vi "Write Interface Infos.vi"(8 "error in (no error)":errorcluster, 10 "Interface Infos":T1, 11 "Application in":refnum<class "Application.lvclass">) -> (0 "error out":errorcluster, 3 "Application out":refnum<class "Application.lvclass">)   [LabVIEW 2018, in "Application.lvclass"]
uses:
  Application.lvclass
  Application.lvclass/Application.ctl
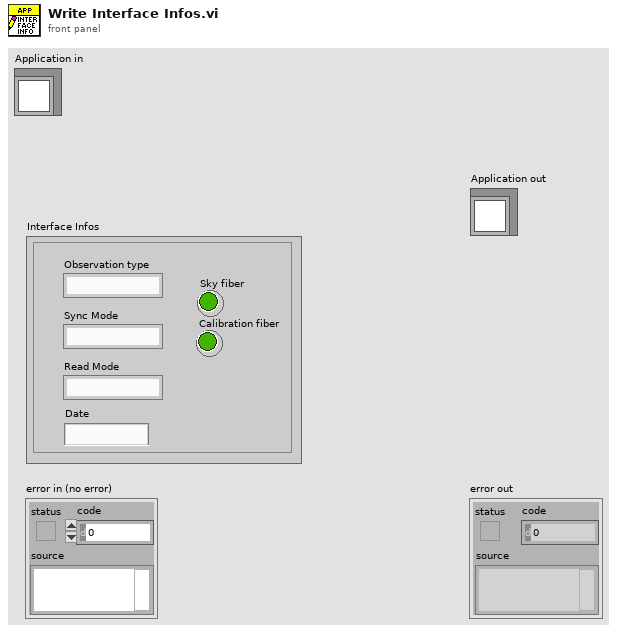
[diagram p1: front panel]
types:
  T1 = cluster{"Observation type":string, "Read Mode":string, "Sky fiber":bool, "Calibration fiber":bool, "Sync Mode":string, "Date":string}
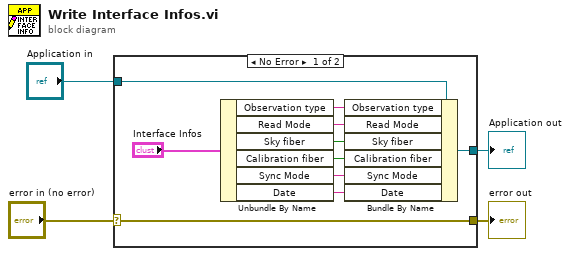
[diagram p0: block diagram]
diagram:
  n1 = case shown="No Error" "error in (no error)" {
    selector: "error in (no error)" -> [w14 w15]
    tunnel: [w14 w15] -> w3
    tunnel: [w12 w16] -> w1
    tunnel: "Application in" -> [w13 w16]
    frame No Error {
      n2 = Unbundle By Name("Interface Infos") -> ("Observation type"=w5:string, "Read Mode"=w6:string, "Sky fiber"=w7:bool, "Calibration fiber"=w8:bool, "Sync Mode"=w10:string, "Date"=w9:string)
      n3 = Bundle By Name(cluster=w13, "Observation type"=w5, "Read Mode"=w6, "Sky fiber"=w7, "Calibration fiber"=w8, "Sync Mode"=w10, "Date"=w9) -> (w12:refnum<class "Application.lvclass">)
    }
    frame Error {
    }
  }
  "error out" <- w3
  "Application out" <- w1
